vi "projektsemLABVIEW.vi"() -> ()   [LabVIEW 2025]
panel:
  out "estymator nieobciazany wariancji":dbl
  out "odchylenie standardowe":dbl
  out "arytm":dbl
  in  "Sample rate (Hz)":dbl=48000.0
  in  "zabezpiecznie":i32
  out "dominujaca czestotliwosc":dbl
  in  "10 \"A\"":dbl[](array[numeric])
  in  "czas (s)":dbl=1.0 caption="Duration (s)"
  out "Widmo amplitudowe":waveform(dbl)(graph)
  out "Spektrum mocy":waveform(dbl)(graph)
  out "Gêstoœæ widmowa mocy":waveform(dbl)(graph)
  out "Gêtoœæ widmowa energii":waveform(dbl)(graph)
  out "moc P":dbl
  out "energia E":dbl
  out "Przebieg czasowy":waveform(dbl)(graph)
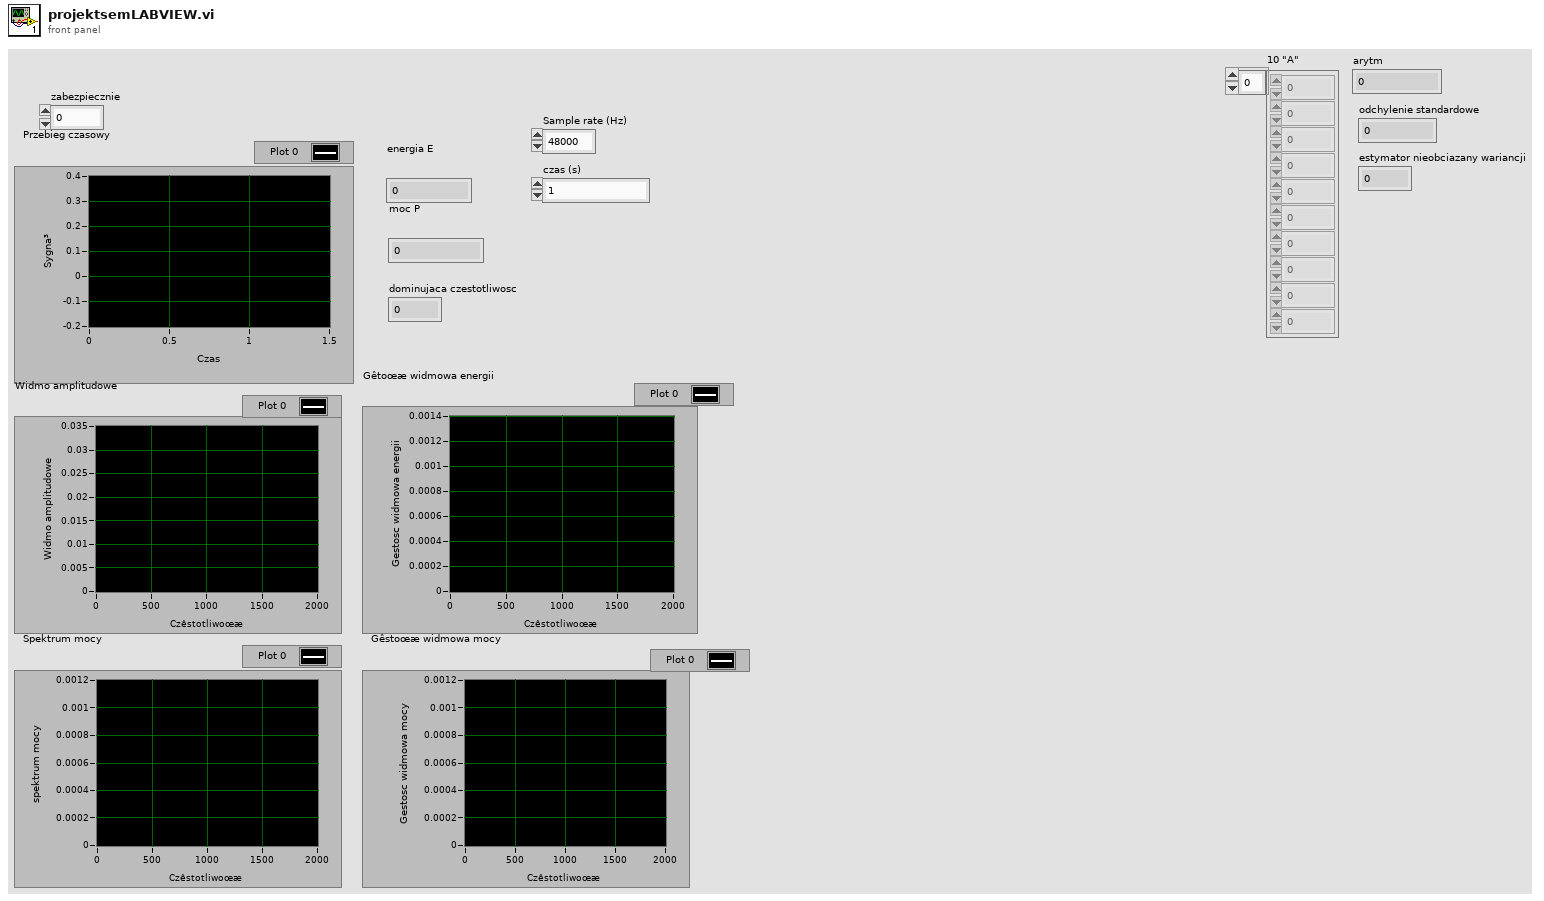
[diagram p1: front panel]
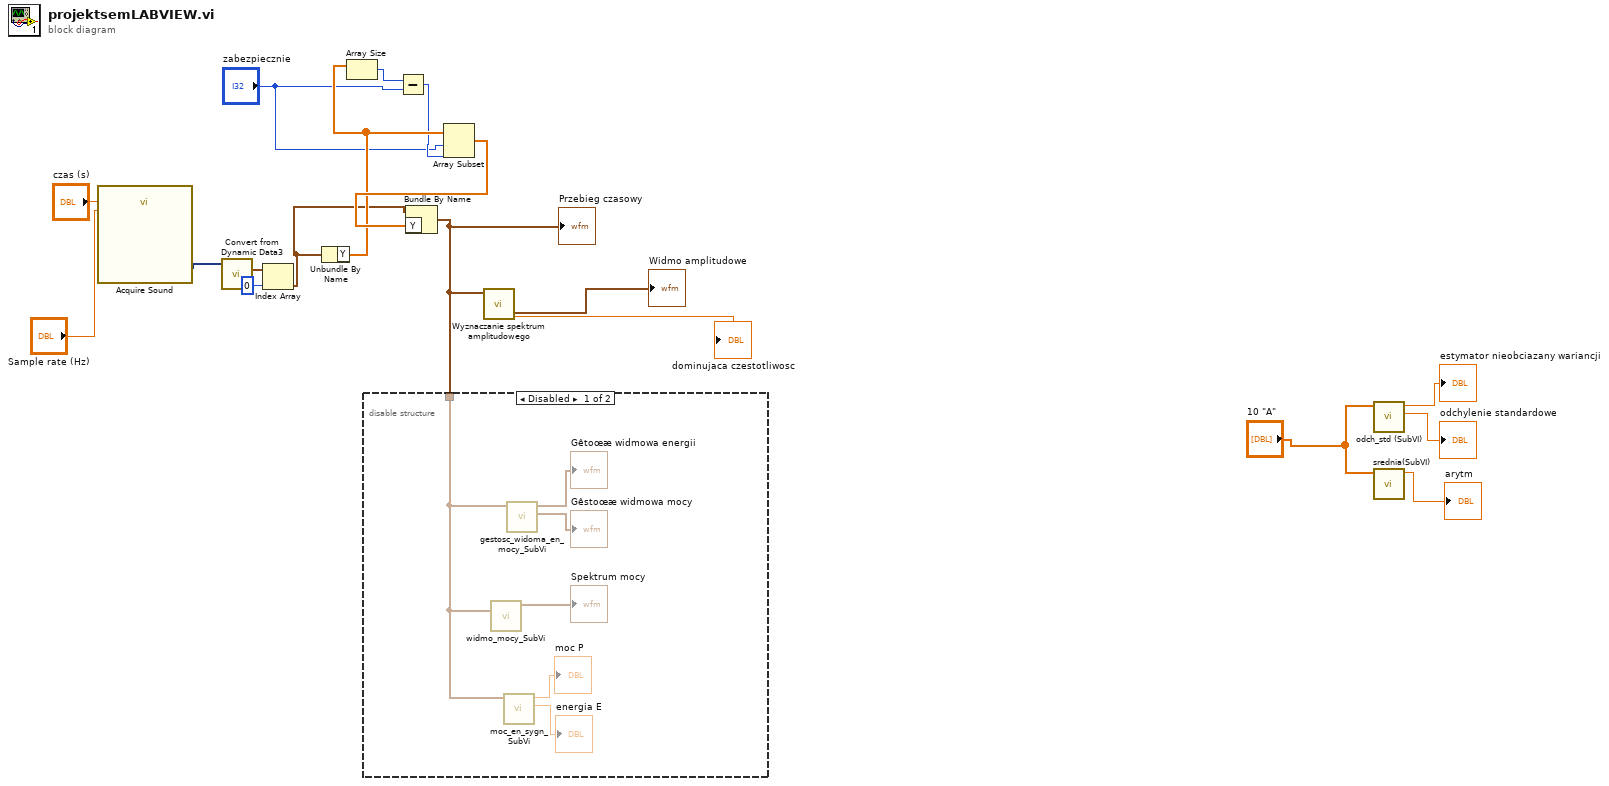
[diagram p0: block diagram]
diagram:
  n1 = call "Acquire Sound"("Duration (s)"="czas (s)", "Sample rate (Hz)"="Sample rate (Hz)") -> ("Data"=w13:dynamicdata)  [unwired: 16 in, 1 out]
  n2 = call "Convert from Dynamic Data3"("Dynamic Data Type"=w13) -> ("Array of Waveform"=w11:waveform(dbl)[])  [unwired: 3 in]
  n3 = Index Array(array=w11, index=0) -> (element=w6:waveform(dbl))
  n4 = Unbundle By Name(w6) -> ("Y"=w12:dbl[])
  n5 = Array Size(array=w12) -> (size(s)=w15:i32)
  n6 = Subtract(x=w15, y="zabezpiecznie") -> (x-y=w9:i32)
  n7 = Array Subset(array=w12, index="zabezpiecznie", length=w9) -> (w14:dbl[])
  n8 = Bundle By Name(cluster=w6, "Y"=w14) -> (w10:waveform(dbl))
  "Przebieg czasowy" <- w10
  n9 = disable-structure shown="Disabled" {
    disable-tunnel: w10 -> [w19 _]
    frame Disabled {
      n10 = call "widmo_mocy_SubVi.vi"("signal in"=w19) -> ("widmo mocy"=→"Spektrum mocy":waveform(dbl))  [unwired: 10 in]
      n11 = call "moc_en_sygn_SubVi.vi"("signal in"=w19) -> ("energia"=→"energia E":dbl, "Moc sygn okr"=→"moc P":dbl)  [unwired: 9 in]
      n12 = call "gestosc_widoma_en_mocy_SubVi.vi"("signal in"=w19) -> ("gestosc widmowa mocy"=→"Gêstoœæ widmowa mocy":waveform(dbl), "gestosc widmowa energii"=→"Gêtoœæ widmowa energii":waveform(dbl))  [unwired: 9 in]
    }
    frame Enabled {
    }
  }
  n13 = call "Wyznaczanie spektrum amplitudowego.vi"("signal in"=w10) -> ("dominujaca czestotliwosc"=→"dominujaca czestotliwosc":dbl, "Waveform"=→"Widmo amplitudowe":waveform(dbl))  [unwired: 4 in, 5 out]
  n14 = call "odch_std (SubVI).vi"("Gaussian noise pattern"="10 \"A\"") -> ("odchylenie standardowe"=→"odchylenie standardowe":dbl, "estymator nieobciazany wariancji"=→"estymator nieobciazany wariancji":dbl)  [unwired: 9 in]
  n15 = call "srednia(SubVI).vi"("input"="10 \"A\"") -> ("arytm"=→"arytm":dbl)  [unwired: 8 in, 2 out]
